vi "SinXsinY Func.vi"(10 "Y length":i32, 11 "X length":i32) -> (1 "Z":dbl[][](array[numeric]), 2 "Y Out":dbl[](array[numeric]), 3 "X Out":dbl[](array[numeric]))   [LabVIEW 2023]
doc: "Generate a surface model of the sin(x)*sin(y) function."
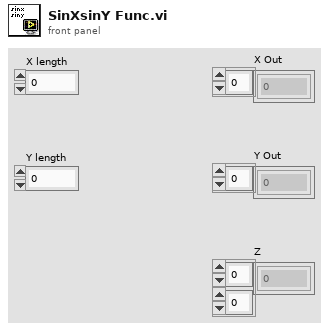
[diagram p1: front panel]
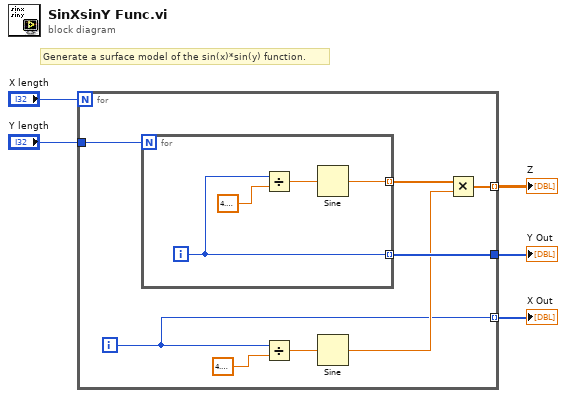
[diagram p0: block diagram]
diagram:
  # "Generate a surface model of the sin(x)*sin(y) function."
  n1 = for {
    N: "X length" -> [_]
    tunnel: [w13] -> w2
    tunnel: [w8] -> w1 mode=indexing
    tunnel: [w7] -> w3 mode=indexing
    tunnel: "Y length" -> [w6]
    i -> [w7]
    n2 = for {
      N: w6 -> [_]
      tunnel: [w15] -> w10 mode=indexing
      tunnel: [w14] -> w13 mode=indexing
      i -> [w14]
      n3 = Divide(x=w14, y=sgl 4.2) -> (x/y=w16:sgl)
      n4 = Sine(x=w16) -> (sin(x)=w15:sgl)
    }
    n5 = Divide(x=w7, y=sgl 4.2) -> (x/y=w12:sgl)
    n6 = Sine(x=w12) -> (sin(x)=w9:sgl)
    n7 = Multiply(x=w10, y=w9) -> (x*y=w8:sgl[])
  }
  "Z" <- w1
  "X Out" <- w3
  "Y Out" <- w2
